vi "Write Search.vi"(10 "Search.lvclass":refnum<class "Search.lvclass">, 11 "DiagramObject in":refnum<class "GObject.lvclass">) -> (3 "DiagramObject out":refnum<class "GObject.lvclass">)   [LabVIEW 2016, in "GObject.lvclass"]
uses:
  GObject.lvclass
  Search/Search.lvclass
  GObject.lvclass/GObject.ctl
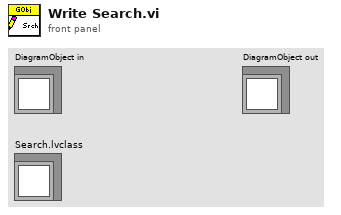
[diagram p1: front panel]
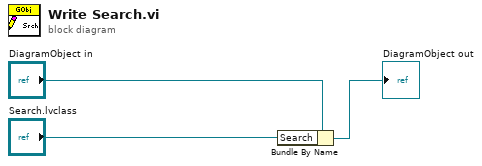
[diagram p0: block diagram]
diagram:
  n1 = Bundle By Name(cluster="DiagramObject in", "Search"="Search.lvclass") -> (→"DiagramObject out":refnum<class "GObject.lvclass">)
